vi "Close Session.vi"(8 "error in":errorcluster, 11 "session In":T1) -> (0 "error out":errorcluster)   [LabVIEW 2023]
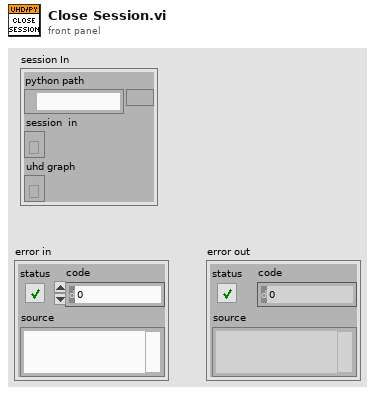
[diagram p1: front panel]
types:
  T1 = cluster{"python path":path, "session  in":refnum<k35>, "uhd graph":refnum<k38>}
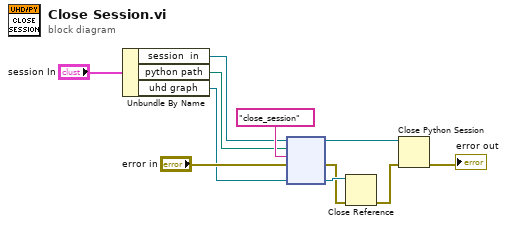
[diagram p0: block diagram]
diagram:
  n1 = Unbundle By Name("session In") -> ("session  in"=w1:refnum<k35>, "python path"=w2:path, "uhd graph"=w3:refnum<k38>)
  n2 = node(w1, w2, "close_session" ("function name"), "error in", w3) -> (w6:refnum<k35>, w8:errorcluster, w9:refnum<k38>)  [unwired: 2 in, 2 out]
  n3 = Close Reference(reference=w9, error in (no error)=w8) -> (error out=w7:errorcluster)
  n4 = Close Python Session(session in=w6, error in=w7) -> (11:→"error out":errorcluster)
